vi "PDLM_GetTagValueList.vi"(8 "error in (no error)":errorcluster, 10 "TaggedValueList":T1 {"Tag" format="%x" items=["NONE"=0, "Locked"=16, "SoftLock"=17, "KeyLock"=18, "Class_IV_Lock"=20, "Interlock"=24, "LaserMode"=32, "LDH_PulsePowerTable"=33, "TriggerMode"=48, "TriggerLevelRaw"=64, "TriggerLevelRawLoLimit"=65, "TriggerLevelRawHiLimit"=66, "TriggerLevel"=72, "TriggerLevelLoLimit"=73, "TriggerLevelHiLimit"=74, "FastGate"=80, "FastGateImp"=96, "SlowGate"=112, "TargetTempRaw"=144, "TargetTempRawLoLimit"=145, "TargetTempRawHiLimit"=146, "CurrentTempRaw"=148, "CaseTempRaw"=149, "TargetTemp"=152, "TargetTempLoLimit"=153, "TargetTempHiLimit"=154, "CurrentTemp"=156, "CaseTemp"=157, "TempScale"=159, "Frequency"=168, "FrequencyLoLimit"=169, "FrequencyHiLimit"=170, "PulsePowerRaw"=176, "PulsePowerRawLoLimit"=177, "PulsePowerRawHiLimit"=178, "PulsePowerPermille"=180, "PulseShape"=181, "PulsePower"=184, "PulsePowerLoLimit"=185, "PulsePowerHiLimit"=186, "PulsePowerNanowatt"=188, "PulsePowerVoltage"=190, "PulseEnergy"=191, "CwPowerRaw"=192, "CwPowerRawLoLimit"=193, "CwPowerRawHiLimit"=194, "CwPowerPermille"=196, "CwPower"=200, "CwPowerLoLimit"=201, "CwPowerHiLimit"=202, "CwPowerMicroWatt"=204, "BurstLen"=208, "BurstPeriod"=224, "LDH_Fan"=240, "UI_Exclusive"=256]}, 11 "USBIdx":i32) -> (0 "error out":errorcluster, 2 "TaggedValueList out":T1 {"Tag" format="%x" items=["NONE"=0, "Locked"=16, "SoftLock"=17, "KeyLock"=18, "Class_IV_Lock"=20, "Interlock"=24, "LaserMode"=32, "LDH_PulsePowerTable"=33, "TriggerMode"=48, "TriggerLevelRaw"=64, "TriggerLevelRawLoLimit"=65, "TriggerLevelRawHiLimit"=66, "TriggerLevel"=72, "TriggerLevelLoLimit"=73, "TriggerLevelHiLimit"=74, "FastGate"=80, "FastGateImp"=96, "SlowGate"=112, "TargetTempRaw"=144, "TargetTempRawLoLimit"=145, "TargetTempRawHiLimit"=146, "CurrentTempRaw"=148, "CaseTempRaw"=149, "TargetTemp"=152, "TargetTempLoLimit"=153, "TargetTempHiLimit"=154, "CurrentTemp"=156, "CaseTemp"=157, "TempScale"=159, "Frequency"=168, "FrequencyLoLimit"=169, "FrequencyHiLimit"=170, "PulsePowerRaw"=176, "PulsePowerRawLoLimit"=177, "PulsePowerRawHiLimit"=178, "PulsePowerPermille"=180, "PulseShape"=181, "PulsePower"=184, "PulsePowerLoLimit"=185, "PulsePowerHiLimit"=186, "PulsePowerNanowatt"=188, "PulsePowerVoltage"=190, "PulseEnergy"=191, "CwPowerRaw"=192, "CwPowerRawLoLimit"=193, "CwPowerRawHiLimit"=194, "CwPowerPermille"=196, "CwPower"=200, "CwPowerLoLimit"=201, "CwPowerHiLimit"=202, "CwPowerMicroWatt"=204, "BurstLen"=208, "BurstPeriod"=224, "LDH_Fan"=240, "UI_Exclusive"=256]}, 3 "return type":i32)   [LabVIEW 2019]
uses:
  <userlib>/TaikoLaser/PDLM_TaggedValueList.ctl
  <userlib>/TaikoLaser/PDLM_TaggedValue.ctl
  <userlib>/TaikoLaser/PDLM_Tag.ctl
  <userlib>/TaikoLaser/PDLM_DllPath_global.vi
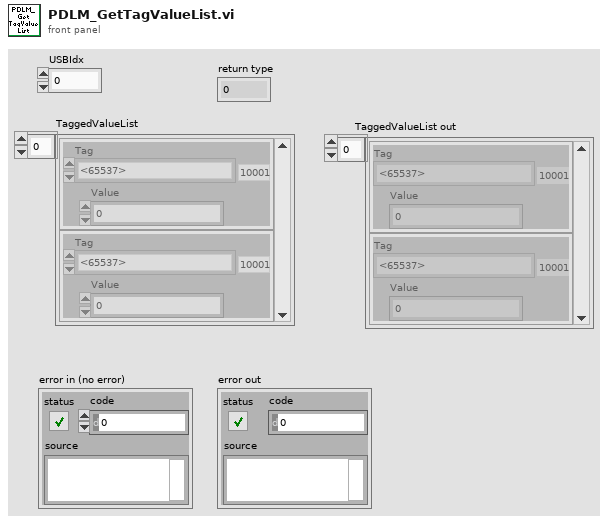
[diagram p1: front panel]
types:
  T1 = typedef "PDLM_TaggedValueList.ctl" = T2[]
  T2 = typedef "PDLM_TaggedValue.ctl" = cluster{"Tag":T3, "Value":u32}
  T3 = typedef "PDLM_Tag.ctl" = u32
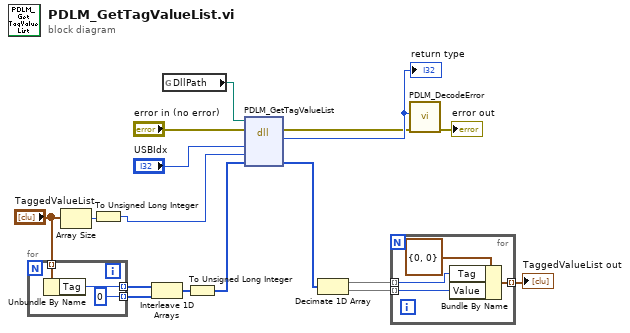
[diagram p0: block diagram]
diagram:
  n1 = for {
    tunnel: "TaggedValueList" -> [w20] mode=indexing
    tunnel: [u32 0] -> w9 mode=indexing
    tunnel: [w18] -> w8 mode=indexing
    n2 = Unbundle By Name(w20) -> ("Tag"=w18:T3)
  }
  n3 = Array Size(array="TaggedValueList") -> (size(s)=w11:i32)
  n4 = To Unsigned Long Integer(number=w11) -> (unsigned 32bit integer=w5:u32)
  n5 = Interleave 1D Arrays(w8, w9) -> (w7:T3[])
  n6 = global read "PDLM_DllPath_global.vi" "DllPath"() -> (w13:path)
  n7 = To Unsigned Long Integer(number=w7) -> (unsigned 32bit integer=w6:T3[])
  n8 = dll-call lib="M:/_dev/progs/LabVIEW/_lib/PQ/Taiko/pdlm_lib.dll" fn="PDLM_GetTagValueList"(path in=w13, error in="error in (no error)", "USBIdx"="USBIdx", "ListLen"=w5, "TagValueList"=w6) -> (error out=w15:errorcluster, "return type"=w16:i32, "TagValueList"=w4:u32[])  [unwired: 3 in, 1 out]
  "return type" <- w16
  n9 = Decimate 1D Array(w4) -> (w3:u32[], w2:u32[])
  n10 = for {
    tunnel: w3 -> [w23] mode=indexing
    tunnel: w2 -> [w22] mode=indexing
    tunnel: [w21] -> w1 mode=indexing
    n11 = Bundle By Name(cluster=T2 {"Tag"=0, "Value"=0} ("TaggedValue"), "Tag"=w23, "Value"=w22) -> (w21:T2)
  }
  "TaggedValueList out" <- w1
  n12 = call <userlib>:"PDLM_DecodeError.vi"("error in (no error)"=w15, "code"=w16) -> ("error out"=→"error out":errorcluster)  [unwired: 7 in, 2 out]
